vi "PBKDF2 Hash.vi"(8 "error in (no error)":errorcluster, 11 "password":string) -> (0 "error out":errorcluster, 2 "salt":string, 3 "hash":string)   [LabVIEW 2013]
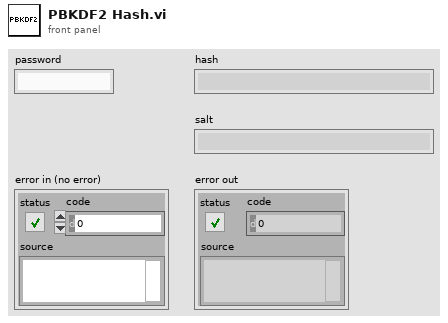
[diagram p1: front panel]
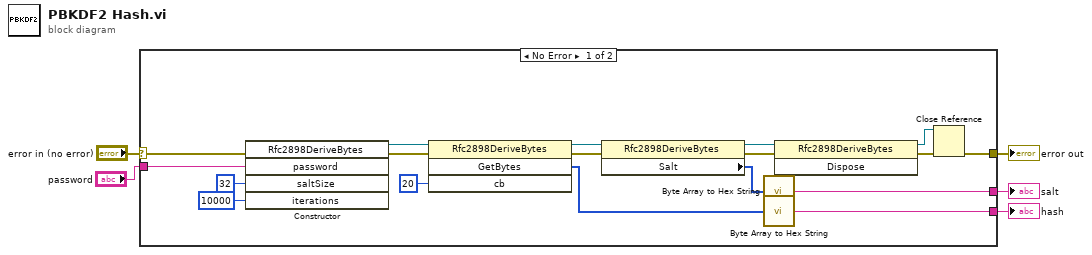
[diagram p0: block diagram]
diagram:
  n1 = case shown="No Error" "error in (no error)" {
    selector: "error in (no error)" -> [w15 w24]
    tunnel: "password" -> [w21 _]
    tunnel: [w12 _] -> w4
    tunnel: [w14 w24] -> w2
    tunnel: [w6 _] -> w1
    frame No Error {
      n2 = constructor class="Rfc2898DeriveBytes" ("k1")(error in=w15, "password"=w21, "saltSize"=32, "iterations"=10000 ("MyIterations")) -> (reference out=w23:refnum<k24>, error out=w22:errorcluster)  [unwired: 2 in, 4 out]
      n3 = invoke class="Rfc2898DeriveBytes" method="GetBytes"(reference=w23, error in=w22, "cb"=20) -> (reference out=w9:refnum<k24>, error out=w18:errorcluster, "GetBytes"=w13:u8[])  [unwired: 1 in, 1 out]
      n4 = property class="Rfc2898DeriveBytes"(reference=w9, error in=w18) -> (reference out=w8:refnum<k24>, error out=w10:errorcluster, "Salt"=w7:u8[])
      n5 = call "Byte Array to Hex String.vi"("bytes array"=w7) -> ("hex string"=w6:string)
      n6 = call "Byte Array to Hex String.vi"("bytes array"=w13) -> ("hex string"=w12:string)
      n7 = invoke class="Rfc2898DeriveBytes" method="Dispose"(reference=w8, error in=w10) -> (reference out=w16:refnum<k24>, error out=w17:errorcluster)  [unwired: 1 in, 1 out]
      n8 = Close Reference(reference=w16, error in (no error)=w17) -> (error out=w14:errorcluster)
    }
    frame Error {
    }
  }
  "hash" <- w4
  "error out" <- w2
  "salt" <- w1
